vi "Parse qKLS type answer by type.vi"(0 "KLS? response":string, 1 "Type":string, 5 "error in (no error)":errorcluster) -> (14 "Names":string[](array[string]), 19 "error out":errorcluster)   [LabVIEW 2026]
doc: "Filters the response of KLS? type answers by the selected type and returns all names related to that type."
uses:
  <vilib>/regexp/Match Regular Expression.xnode
panel:
  # "Filters the response of KLS? type answers by the selected type\nand returns all names related to that type."
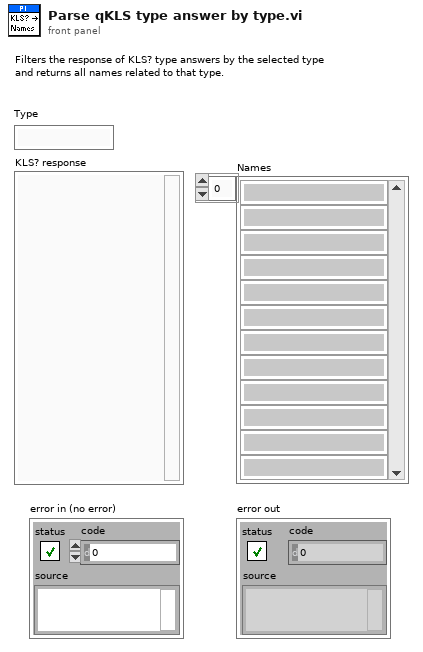
[diagram p1: front panel]
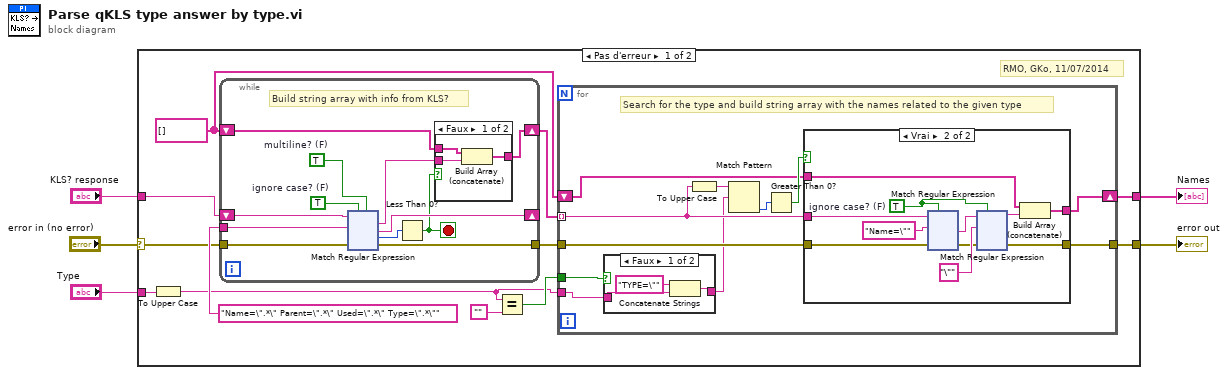
[diagram p0: block diagram]
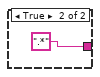
[diagram p2: hidden frame]
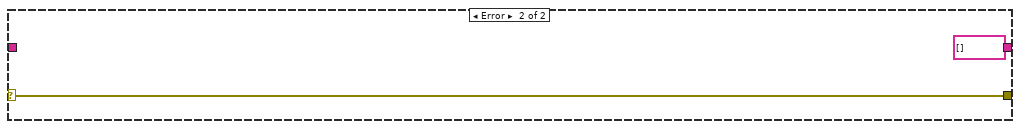
[diagram p5: hidden frame]
diagram:
  n1 = case shown="Pas d'erreur" "error in (no error)" {
    selector: "error in (no error)" -> [w12 w414]
    tunnel: [w15 string[] []] -> w5
    tunnel: "KLS? response" -> [w13 _]
    tunnel: [w10 w414] -> w3
    tunnel: "Type" -> [w7 _]
    frame No Error {
      w14 = string[] []
      # "RMO, GKo, 11/07/2014"
      n2 = To Upper Case(1:w7) -> (0:w6:string)
      n3 = while {
        shift-right: [w286] -> _
        shift-left: w13 -> [w289]
        tunnel: "Name=\".*\" Parent=\".*\" Used=\".*\" Type=\".*\"" -> [w283]
        shift-right: [w285] -> w16
        shift-left: w14 -> [w288]
        tunnel: w12 -> [w281]
        tunnel: [w280] -> w11
        stop <- w282 stop-if-true
        w291 = TRUE  # ignore case? (F)
        w290 = TRUE  # multiline? (F)
        # "Build string array with info from KLS?"
        n4 = xnode "Match Regular Expression"("chaîne en entrée"=w289, "expression régulière"=w283, "entrée d'erreur"=w281, "ignorer la casse ? (F)"=w291, "multiligne ? (F)"=w290) -> ("toute l'expression"=w287:string, "après la correspondance"=w286:string, "offset après correspondance"=w284:i32, "sortie d'erreur"=w280:errorcluster)  [unwired: 1 in, 1 out]
        n5 = Less Than 0?(x=w284) -> (x < 0?=w282:bool)
        n6 = case shown="Faux" w282 {
          tunnel: w288 -> [w294 w295]
          tunnel: w287 -> [w293 _]
          tunnel: [w292 w295] -> w285
          frame False {
            n7 = Build Array (concatenate)(w294, w293) -> (w292:string[])
          }
          frame True {
          }
        }
      }
      n8 = Equal?(x=w6, y="") -> (x = y?=w9:bool)
      n9 = for {
        tunnel: w16 -> [w22] mode=indexing
        shift-right: [w25] -> w15
        shift-left: w14 -> [w26]
        tunnel: w11 -> [w24]
        tunnel: [w23] -> w10
        tunnel: w9 -> [w19]
        tunnel: w6 -> [w18]
        # "Search for the type and build string array with the names related to the given type"
        n10 = case shown="Faux" w19 {
          tunnel: [w29 ".*"] -> w20
          tunnel: w18 -> [w30 _]
          frame False {
            n11 = Concatenate Strings("TYPE=\"", w30) -> (w29:string)
          }
          frame True {
          }
        }
        n12 = To Upper Case(1:w22) -> (0:w21:string)
        n13 = Match Pattern(string=w21, regular expression=w20) -> (offset past match=w28:i32)  [unwired: 4 out]
        n14 = Greater Than 0?(x=w28) -> (x > 0?=w27:bool)
        n15 = case shown="Vrai" w27 {
          tunnel: w22 -> [_ w41]
          tunnel: w26 -> [w34 w40]
          tunnel: [w34 w38] -> w25
          tunnel: w24 -> [w33 w37]
          tunnel: [w33 w35] -> w23
          frame False {
          }
          frame True {
            w44 = TRUE  # ignore case? (F)
            n16 = xnode "Match Regular Expression"("chaîne en entrée"=w41, "expression régulière"="Name=\"", "entrée d'erreur"=w37, "ignorer la casse ? (F)"=w44) -> ("après la correspondance"=w42:string, "sortie d'erreur"=w36:errorcluster)  [unwired: 1 in, 4 out]
            n17 = xnode "Match Regular Expression"("chaîne en entrée"=w42, "expression régulière"="\"", "entrée d'erreur"=w36, "ignorer la casse ? (F)"=w44) -> ("avant la correspondance"=w39:string, "sortie d'erreur"=w35:errorcluster)  [unwired: 1 in, 4 out]
            n18 = Build Array (concatenate)(w40, w39) -> (w38:string[])
          }
        }
      }
    }
    frame Error {
    }
  }
  "Names" <- w5
  "error out" <- w3
